vi "rm.server.set vizualization menu.vi"(8 "error in (no error)":errorcluster, 11 "menu reference in":refnum<k9>) -> (0 "error out":errorcluster, 3 "menu reference out":refnum<k9>)   [LabVIEW 2016, in "RM.Server.lvlib"]
uses:
  RM.Server.lvlib
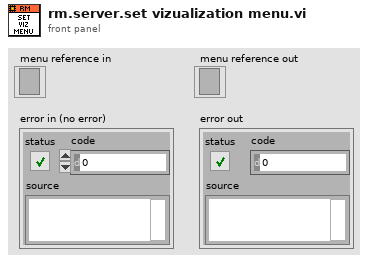
[diagram p1: front panel]
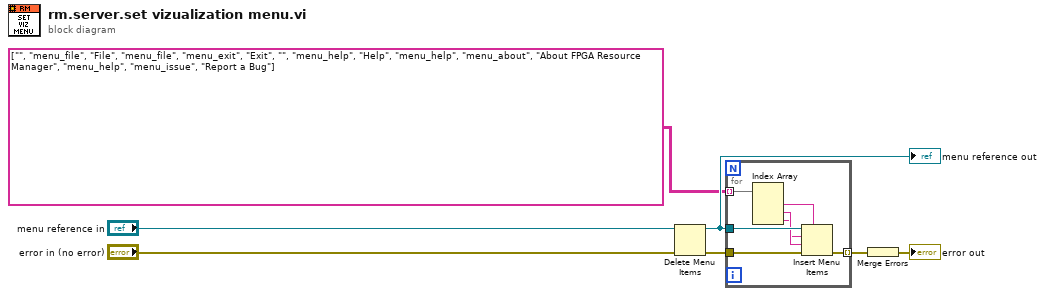
[diagram p0: block diagram]
diagram:
  n1 = Delete Menu Items(6:"error in (no error)", 9:"menu reference in") -> (0:w3:errorcluster, 3:w7:refnum<k9>)  [unwired: 2 in]
  "menu reference out" <- w7
  n2 = for {
    tunnel: string[][] [["", "menu_file", "File"], ["menu_file", "menu_exit", "Exit"], ["", "menu_help", "Help"], ["menu_help", "menu_about", "About FPGA Resource Manager"], ["menu_help", "menu_issue", "Report a Bug"]] -> [w14] mode=indexing
    tunnel: w7 -> [w13]
    tunnel: w3 -> [w11]
    tunnel: [w10] -> w2 mode=indexing
    n3 = Index Array(array=w14) -> (element #1=w12:string, element #2=w9:string, element #3=w8:string)  [unwired: 3 in]
    n4 = Insert Menu Items(5:w12, 6:w11, 7:w9, 8:w8, 9:w13) -> (0:w10:errorcluster)  [unwired: 1 in, 2 out]
  }
  n5 = Merge Errors(w2) -> (→"error out":errorcluster)
